vi "MC_Visiable_Selections.vi"(8 "error in (no error)":errorcluster, 9 "VisiableSymbols":bool, 11 "MCin":refnum<vi>) -> (0 "error out":errorcluster, 3 "MCout":refnum<vi>)   [LabVIEW 2013]
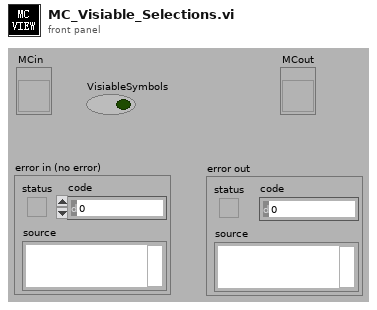
[diagram p1: front panel]
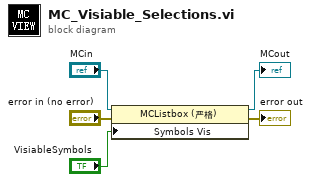
[diagram p0: block diagram]
diagram:
  n1 = property on="属性节点" class="MCListbox (严格)"(reference="MCin", error in="error in (no error)", "Symbols Vis"="VisiableSymbols") -> (reference out=→"MCout":refnum<vi>, error out=→"error out":errorcluster)
